vi "AuMT8852B EDR Maximum Input Power Extended Results.vi"(5 "Stage":T2(ring), 8 "error in (no error)":errorcluster, 11 "VISA session":refnum<visa-resource-name>) -> (0 "error out":errorcluster, 2 "error code":i32, 3 "VISA session out":refnum<visa-resource-name>, 4 "Results":T1 {"3MBs Overall BER" format="%.2e"; "2MBs Overall BER" format="%.2e"})   [LabVIEW 2017]
doc: "Anritsu MT8852B Bluetooth Tester\n\nReturns the results of the EDR Maximum Input Power test.\n\nINPUTS\nStage - results of the individual hopping stages of the test.\n\nOUTPUTS\nResults - measurements made during the test."
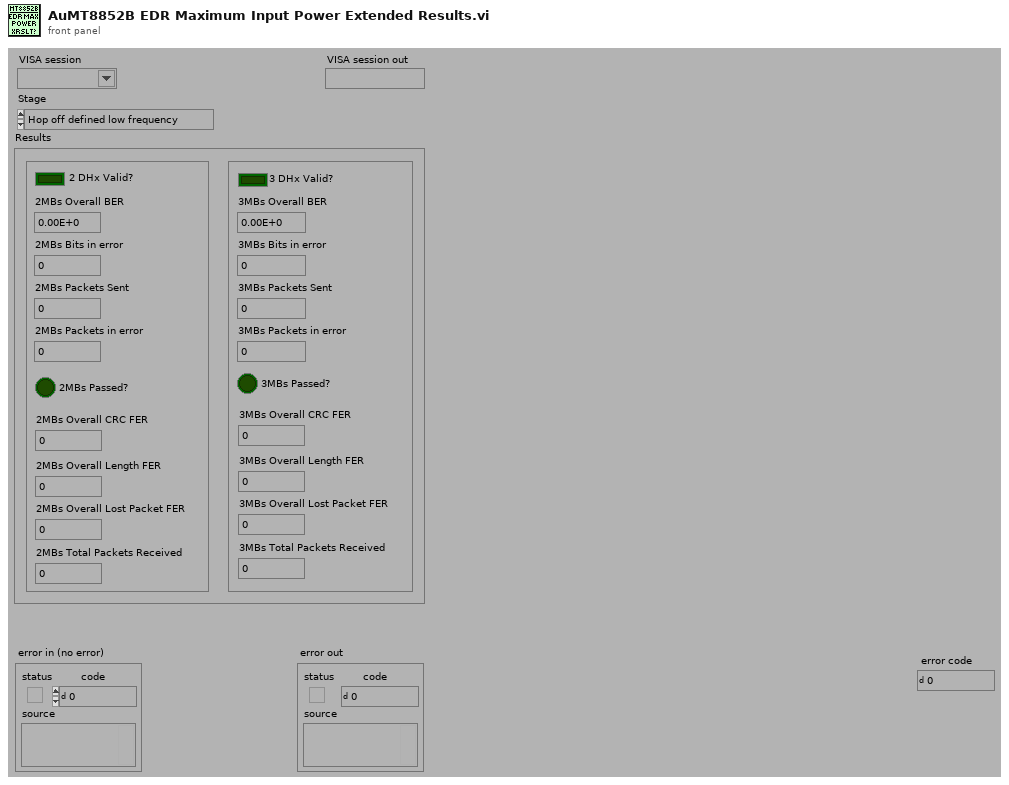
[diagram p1: front panel]
types:
  T1 = cluster{"2 DHx Valid?":bool, "2MBs Overall BER":dbl, "2MBs Bits in error":u32, "2MBs Packets Sent":u32, "2MBs Packets in error":u32, "3 DHx Valid?":bool, "3MBs Overall BER":dbl, "3MBs Bits in error":u32, "3MBs Packets Sent":u32, "3MBs Packets in error":u32, "2MBs Overall CRC FER":u32, "2MBs Overall Length FER":u32, "2MBs Overall Lost Packet FER":u32, "3MBs Overall CRC FER":u32, "3MBs Overall Length FER":u32, "3MBs Overall Lost Packet FER":u32, "2MBs Total Packets Received":u32, "3MBs Total Packets Received":u32, "2MBs Passed?":bool, "3MBs Passed?":bool}
  T2 = enum16{"Hop off defined low frequency", "Hop off defined medium frequency", "Hop off defined high frequency", "Hop on any channels"}
  T3 = enum16{"Simulate", "Range check", "Cache", "Query instrument status"}
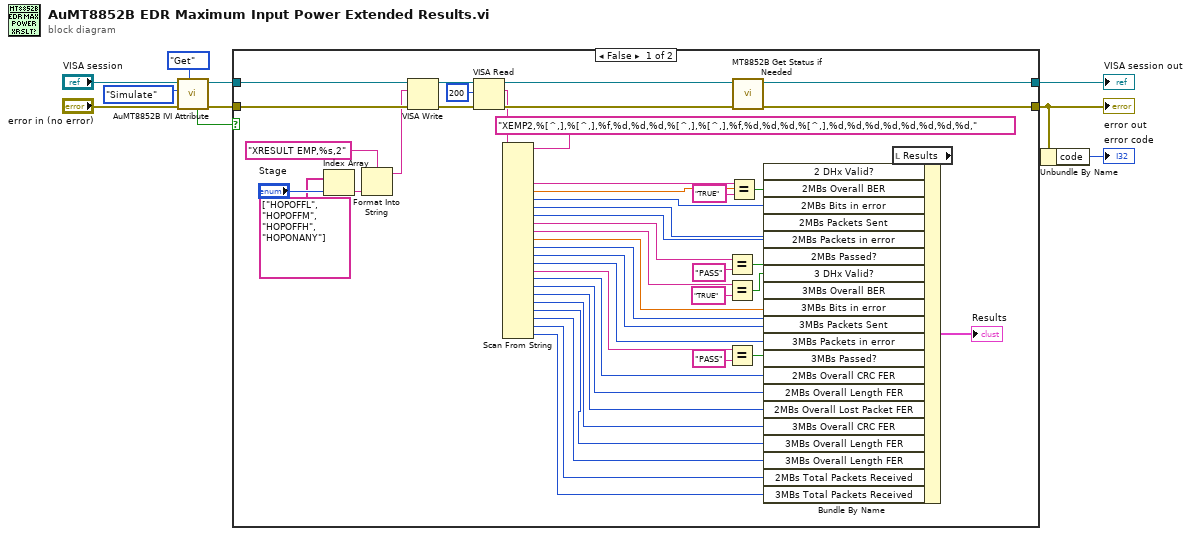
[diagram p0: block diagram]
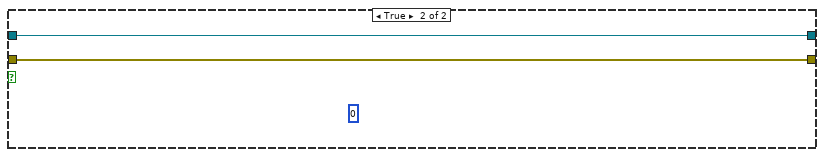
[diagram p2: hidden frame]
diagram:
  n1 = call <instrlib>:"AuMT8852B IVI Attribute.vi"("Set/Get (Set)"=enum16{"Set", "Get"}."Get", "error in (no error)"="error in (no error)", "Flag (Simulate)"=T3."Simulate", "VISA session"="VISA session") -> ("error out"=w7:errorcluster, "VISA session out"=w9:refnum<visa-resource-name>, "Value out"=w3:bool)  [unwired: 5 in]
  n2 = case shown="False" w3 {
    tunnel: [w50 w58] -> w10
    tunnel: [w49 w57] -> w1
    tunnel: w9 -> [w56 w58]
    tunnel: w7 -> [w55 w57]
    frame False {
      n3 = Index Array(array=string[] ["HOPOFFL", "HOPOFFM", "HOPOFFH", "HOPONANY"], index="Stage") -> (element=w38:string)
      n4 = Format Into String(format string="XRESULT EMP,%s,2" ("write buffer (\"\")"), w38) -> (resulting string=w35:string)  [unwired: 2 in, 1 out]
      n5 = VISA Write(VISA resource name=w56, write buffer=w35, error in (no error)=w55) -> (VISA resource name out=w54:refnum<visa-resource-name>, error out=w53:errorcluster)  [unwired: 1 out]
      n6 = VISA Read(VISA resource name=w54, byte count=u32 200 ("byte count (0)"), error in (no error)=w53) -> (VISA resource name out=w48:refnum<visa-resource-name>, read buffer=w33:string, error out=w47:errorcluster)  [unwired: 1 out]
      n7 = Scan From String(format string="XEMP2,%[^,],%[^,],%f,%d,%d,%d,%[^,],%[^,],%f,%d,%d,%d,%[^,],%d,%d,%d,%d,%d,%d,%d,%d," ("Format String"), input string=w33) -> (output 2=w32:string, output 3=w31:dbl, output 4=w30:i32, output 5=w29:i32, output 6=w28:i32, output 7=w27:string, output 8=w26:string, output 9=w25:dbl, output 10=w24:i32, output 11=w23:i32, output 12=w22:i32, output 13=w21:string, output 14=w20:i32, output 15=w19:i32, output 16=w18:i32, output 17=w17:i32, output 18=w16:i32, output 19=w15:i32, output 20=w14:i32, output 21=w13:i32)  [unwired: 24 in, 3 out]
      n8 = Equal?(x=w27, y="PASS") -> (x = y?=w44:bool)
      n9 = Equal?(x=w26, y="TRUE") -> (x = y?=w42:bool)
      n10 = Equal?(x=w21, y="PASS") -> (x = y?=w41:bool)
      n11 = Equal?(x=w32, y="TRUE") -> (x = y?=w46:bool)
      n12 = call <instrlib>:"MT8852B Get Status if Needed.vi"("error in (no error)"=w47, "VISA session"=w48) -> ("error out"=w49:errorcluster, "VISA session out"=w50:refnum<visa-resource-name>)  [unwired: 8 in]
      n13 = local read "Results"() -> (w12:T1)
      n14 = Bundle By Name(cluster=w12, "2 DHx Valid?"=w46, "2MBs Overall BER"=w31, "2MBs Bits in error"=w30, "2MBs Packets Sent"=w29, "2MBs Packets in error"=w28, "2MBs Passed?"=w44, "3 DHx Valid?"=w42, "3MBs Overall BER"=w25, "3MBs Bits in error"=w24, "3MBs Packets Sent"=w23, "3MBs Packets in error"=w22, "3MBs Passed?"=w41, "2MBs Overall CRC FER"=w20, "2MBs Overall Length FER"=w19, "2MBs Overall Lost Packet FER"=w18, "3MBs Overall CRC FER"=w17, "3MBs Overall Length FER"=w16, "3MBs Overall Length FER"=w15, "2MBs Total Packets Received"=w14, "3MBs Total Packets Received"=w13) -> (→"Results":T1)
    }
    frame True {
      (unwired) u8 0
    }
  }
  "error out" <- w1
  "VISA session out" <- w10
  n15 = Unbundle By Name(w1) -> ("code"=→"error code":i32)
